vi "Read database.vi"(5 "String":string) -> (0 "error out":errorcluster, 1 "Operator code":string[](array[string]), 2 "DB Data":T1)   [LabVIEW 2015]
uses:
  <vilib>/addons/database/Connection.llb/DB Tools Open Connec (String).vi
  Galobal variable_TI.vi
  <vilib>/addons/database/_DB Variant To Data/Database Variant To Data.xnode
  <vilib>/addons/database/NI_Database_API.lvlib
panel:
  out "data":string[](array[string])
  out "String 2":string
  out "tables":string[](array[string])
  out "error out 3":errorcluster
  out "appended array 4":string[](array[string])
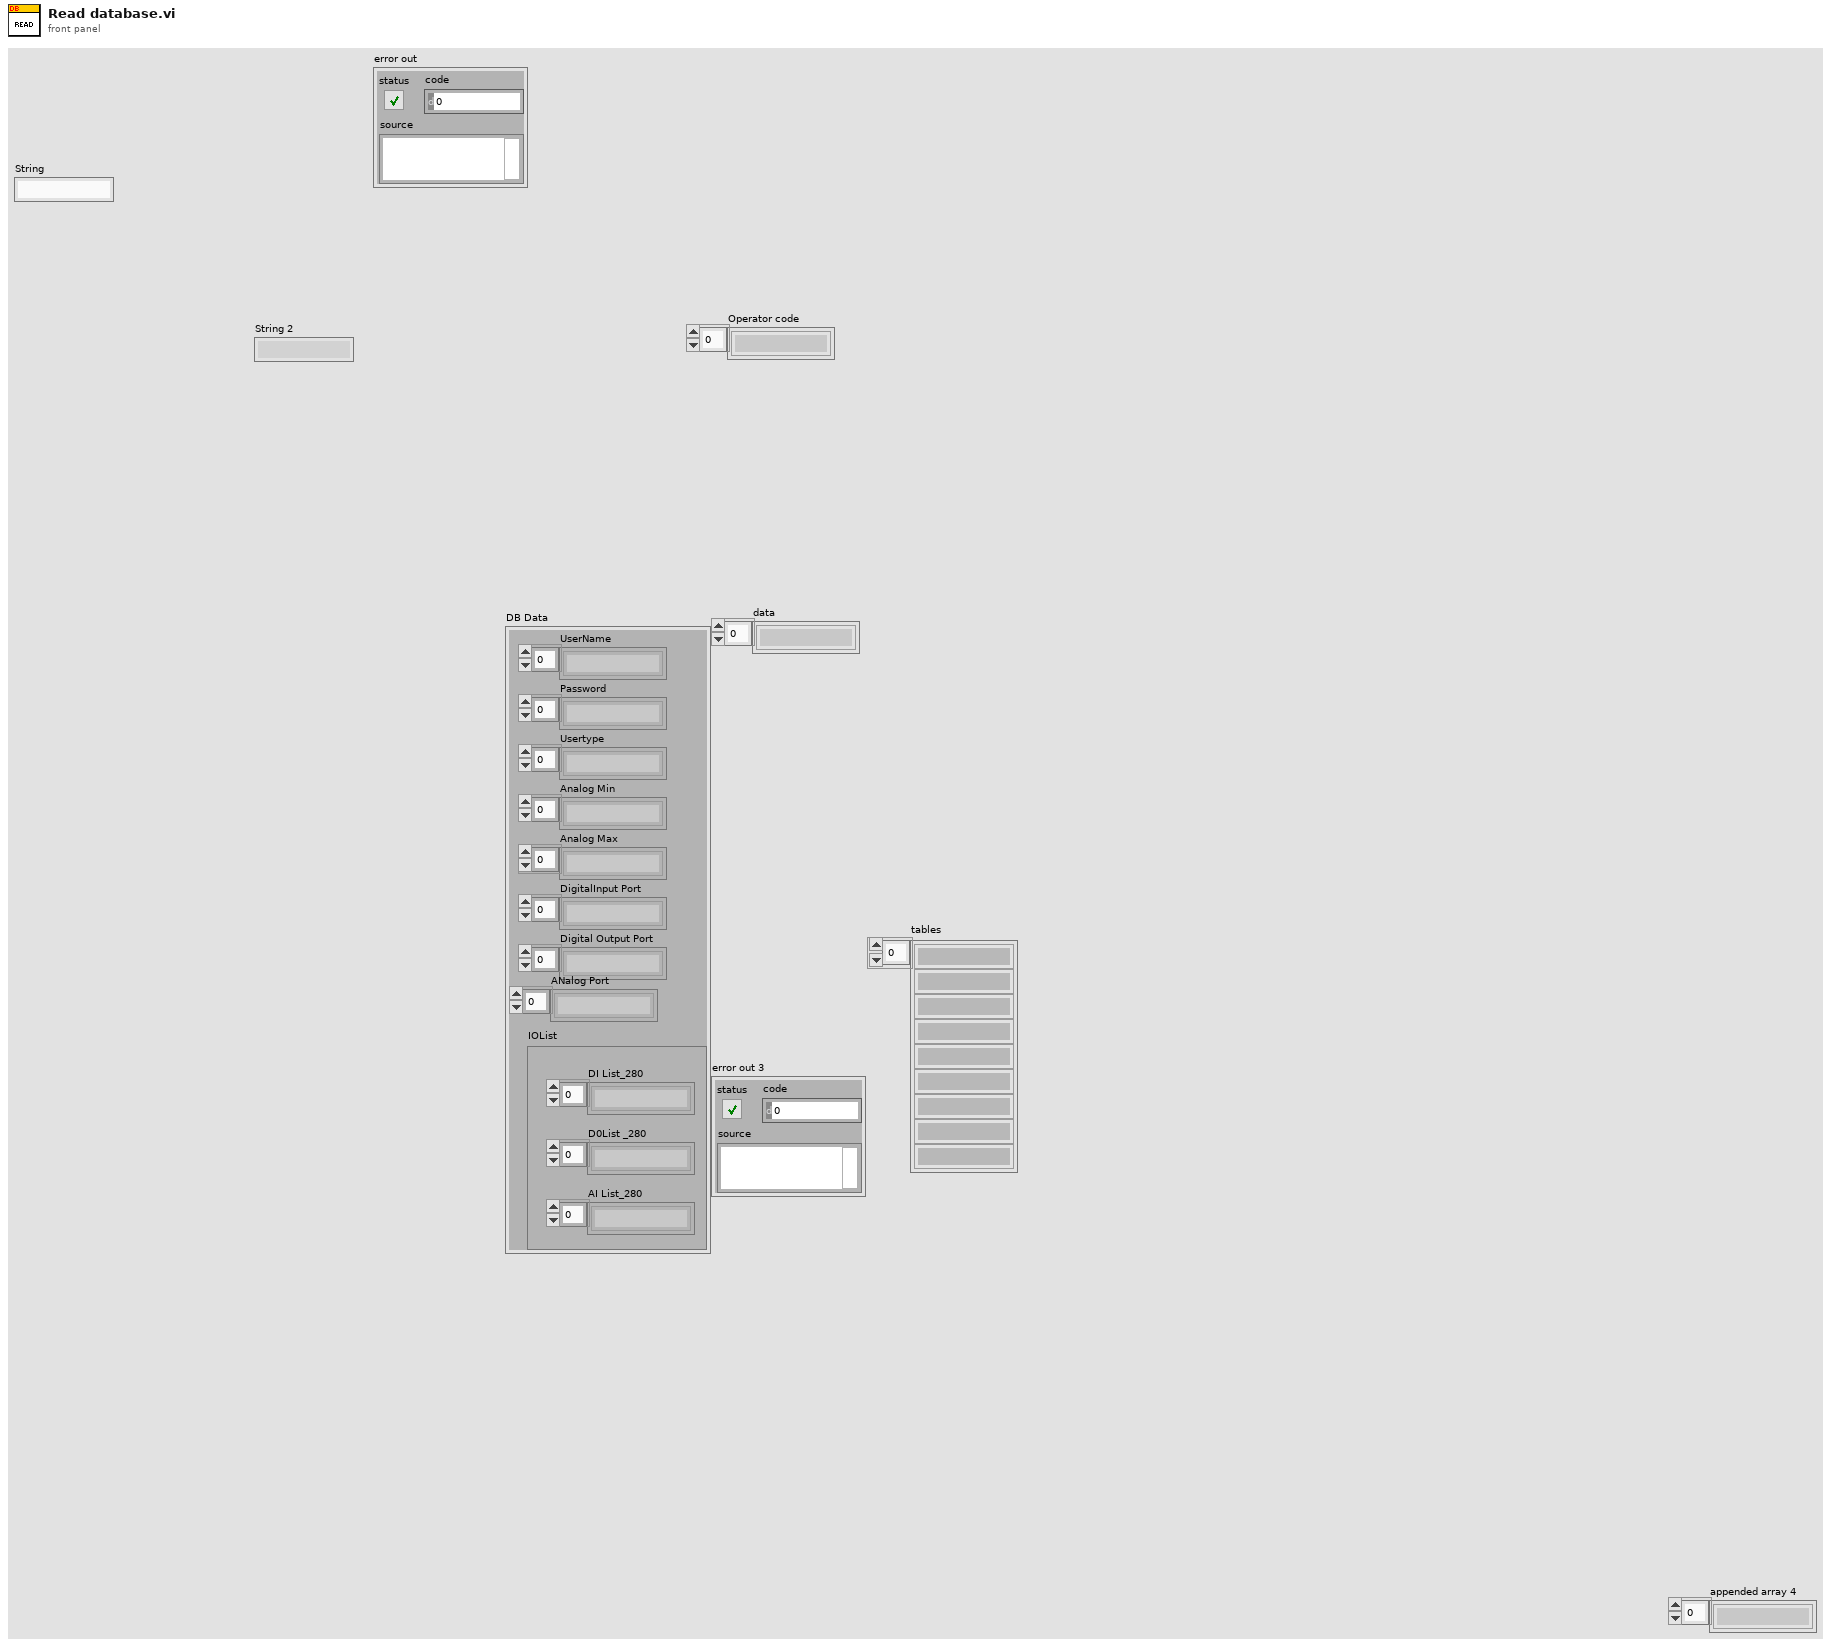
[diagram p1: front panel]
types:
  T1 = cluster{"UserName":string[], "Password":string[], "Usertype":string[], "Analog Min":string[], "Analog Max":string[], "DigitalInput Port":string[], "Digital Output Port":string[], "ANalog Port":string[], "IOList":cluster{"DI List_280":string[], "D0List _280":string[], "AI List_280":string[]}}
  T2 = cluster{"To-A":timestamp, "From-A":timestamp, "From-B":timestamp, "To-B":timestamp, "From-C 1":timestamp, "To-C 1":timestamp, "From-C 2":timestamp, "To-C 2":timestamp, "Shift":string}[]
  T3 = typedef "NI_Database_API.lvlib/Conn ObjectReference.ctl" = refnum<k1>
  T4 = cluster{"DI List_280":string[], "D0List _280":string[], "AI List_280":string[]}
  T5 = cluster{"To-A":timestamp, "From-A":timestamp, "From-B":timestamp, "To-B":timestamp, "From-C 1":timestamp, "To-C 1":timestamp, "From-C 2":timestamp, "To-C 2":timestamp, "Shift":string}
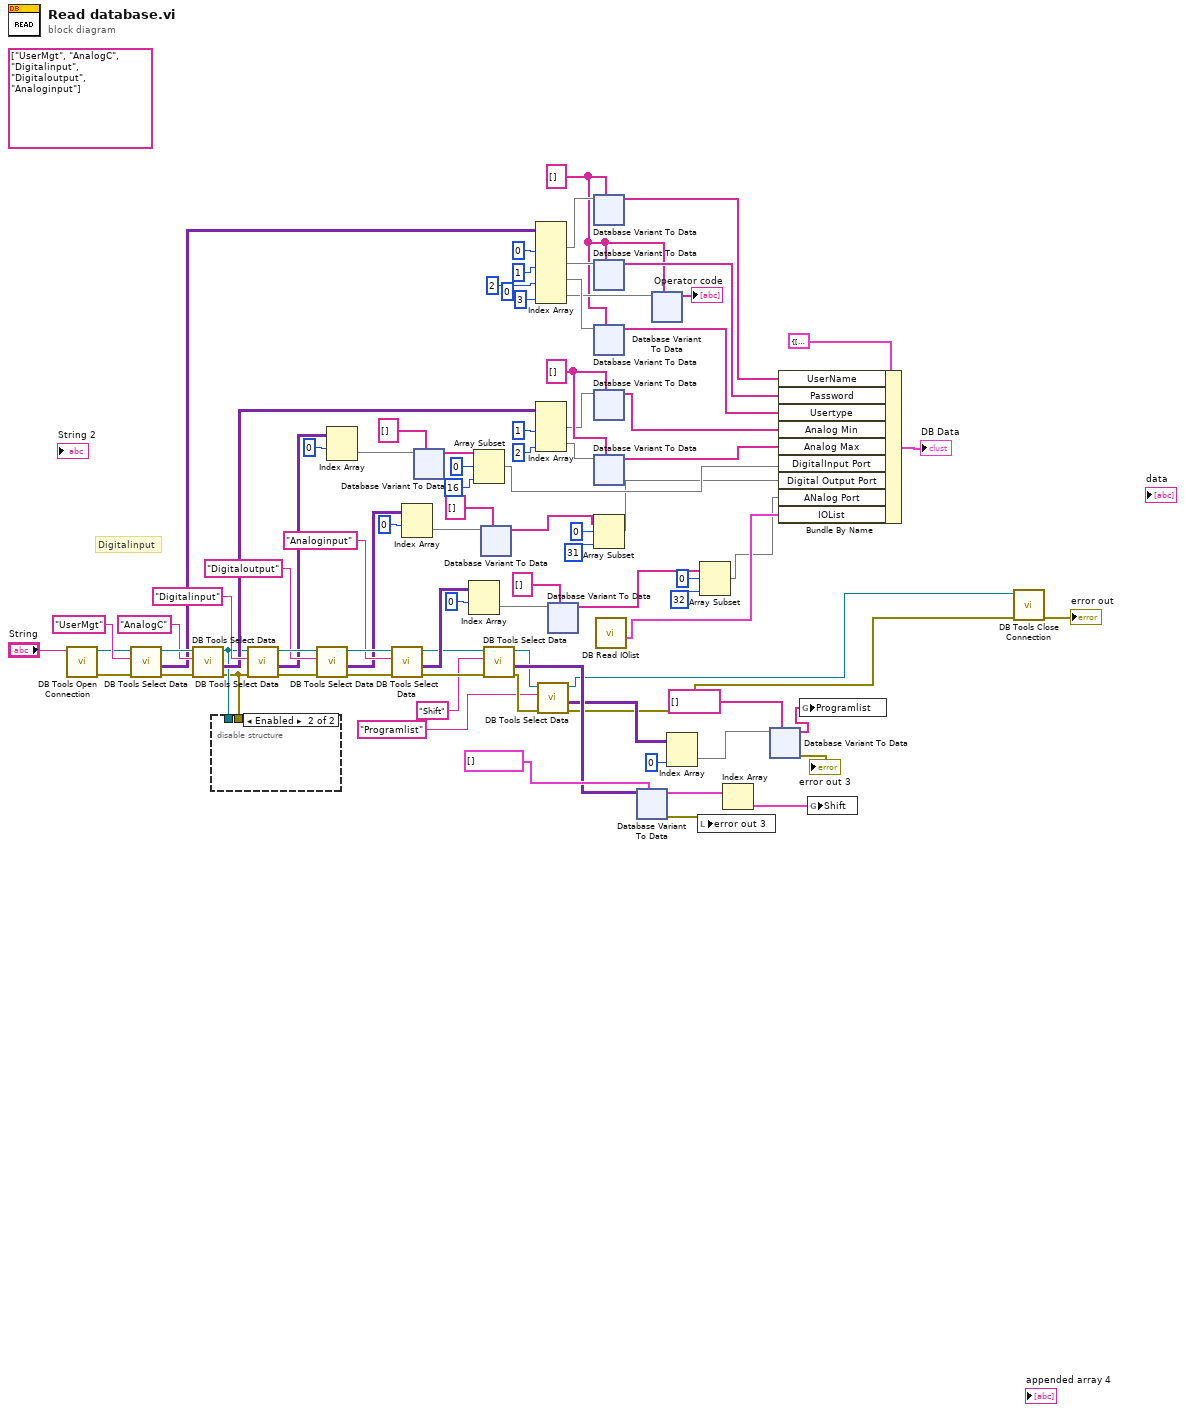
[diagram p0: block diagram]
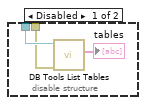
[diagram p2: hidden frame]
diagram:
  (unwired) 0 ("disabled index (row)")
  w76 = string[] []
  (unwired) string[] ["UserMgt", "AnalogC", "Digitalinput", "Digitaloutput", "Analoginput"]
  w2 = string[] []
  # "Digitalinput"
  n1 = call-poly <vilib>:"DB Tools Open Connection.vi"("connection information"="String") -> ("error out"=w46:errorcluster, "connection reference"=w47:T3)  [unwired: 7 in]
  n2 = call <vilib>:"DB Tools Select Data.vi"("error in (no error)"=w46, "table"="UserMgt", "connection reference"=w47) -> ("error out"=w58:errorcluster, "data"=w45:variant[][], "connection reference out"=w57:T3)  [unwired: 3 in]
  n3 = call <vilib>:"DB Tools Select Data.vi"("error in (no error)"=w58, "table"="AnalogC", "connection reference"=w57) -> ("error out"=w8:errorcluster, "data"=w44:variant[][], "connection reference out"=w9:T3)  [unwired: 3 in]
  n4 = disable-structure shown="Enabled" {
    disable-tunnel: w9 -> [w88 _]
    disable-tunnel: w8 -> [w87 _]
    frame Disabled {
      n5 = call <vilib>:"DB Tools List Tables.vi"("error in (no error)"=w87, "connection reference"=w88) -> ("tables"=→"tables":string[])  [unwired: 3 in, 2 out]
    }
    frame Enabled {
    }
  }
  n6 = call <vilib>:"DB Tools Select Data.vi"("error in (no error)"=w8, "table"="Digitalinput", "connection reference"=w9) -> ("error out"=w53:errorcluster, "data"=w43:variant[][], "connection reference out"=w52:T3)  [unwired: 3 in]
  n7 = call <vilib>:"DB Tools Select Data.vi"("error in (no error)"=w53, "table"="Digitaloutput", "connection reference"=w52) -> ("error out"=w49:errorcluster, "data"=w42:variant[][], "connection reference out"=w50:T3)  [unwired: 3 in]
  n8 = Index Array(array=w43, index (row)=0 ("disabled index (col)")) -> (element=w78:variant[])  [unwired: 1 in]
  n9 = call <vilib>:"DB Tools Select Data.vi"("error in (no error)"=w49, "table"="Analoginput", "connection reference"=w50) -> ("error out"=w36:errorcluster, "data"=w41:variant[][], "connection reference out"=w35:T3)  [unwired: 3 in]
  n10 = Index Array(array=w42, index (row)=0 ("disabled index (col)")) -> (element=w79:variant[])  [unwired: 1 in]
  n11 = xnode "Database Variant To Data"("database variant"=w78, "type"=string[] []) -> ("data"=w32:string[])  [unwired: 1 in, 1 out]
  n12 = Index Array(array=w41, index (row)=0 ("disabled index (col)")) -> (element=w82:variant[])  [unwired: 1 in]
  n13 = Array Subset(array=w32, index=0, length=16) -> (w29:string[])
  n14 = xnode "Database Variant To Data"("database variant"=w79, "type"=string[] []) -> ("data"=w27:string[])  [unwired: 1 in, 1 out]
  n15 = call <vilib>:"DB Tools Select Data.vi"("error in (no error)"=w36, "table"="Shift", "connection reference"=w35) -> ("error out"=w19:errorcluster, "data"=w33:variant[][], "connection reference out"=w20:T3)  [unwired: 3 in]
  n16 = Index Array(array=w45, index (col) #1=0 ("disabled index (col)"), index (col) #2=1 ("index (col)"), index (col) #3=2 ("index (col)"), index (col) #4=3 ("index (col)")) -> (element #1=w69:variant[], element #2=w66:variant[], element #3=w65:variant[], element #4=w3:variant[])  [unwired: 4 in]
  n17 = Index Array(array=w44, index (col) #1=1 ("disabled index (col)"), index (col) #2=2 ("index (col)")) -> (element #1=w74:variant[], element #2=w75:variant[])  [unwired: 2 in]
  n18 = call <vilib>:"DB Tools Select Data.vi"("error in (no error)"=w19, "table"="Programlist", "connection reference"=w20) -> ("error out"=w6:errorcluster, "data"=w17:variant[][], "connection reference out"=w7:T3)  [unwired: 3 in]
  n19 = xnode "Database Variant To Data"("database variant"=w82, "type"=string[] []) -> ("data"=w22:string[])  [unwired: 1 in, 1 out]
  n20 = xnode "Database Variant To Data"("database variant"=w69, "type"=w2) -> ("data"=w64:string[])  [unwired: 1 in, 1 out]
  n21 = xnode "Database Variant To Data"("database variant"=w66, "type"=w2) -> ("data"=w63:string[])  [unwired: 1 in, 1 out]
  n22 = xnode "Database Variant To Data"("database variant"=w65, "type"=w2) -> ("data"=w62:string[])  [unwired: 1 in, 1 out]
  n23 = xnode "Database Variant To Data"("database variant"=w74, "type"=w76) -> ("data"=w61:string[])  [unwired: 1 in, 1 out]
  n24 = xnode "Database Variant To Data"("database variant"=w75, "type"=w76) -> ("data"=w60:string[])  [unwired: 1 in, 1 out]
  n25 = Array Subset(array=w27, index=0, length=31) -> (w25:string[])
  n26 = call "DB Read IOlist.vi"() -> ("output cluster"=w21:T4)  [unwired: 11 in]
  n27 = xnode "Database Variant To Data"("database variant"=w33, "type"=T2 []) -> ("data"=w37:T2, "error out"=w10:errorcluster)  [unwired: 1 in]
  n28 = xnode "Database Variant To Data"("database variant"=w3, "type"=w2) -> ("data"=→"Operator code":string[])  [unwired: 1 in, 1 out]
  n29 = Index Array(array=w17, index (col)=0 ("disabled index (col)")) -> (element=w16:variant[])  [unwired: 1 in]
  n30 = local write "error out 3"(w10) -> ()
  n31 = Array Subset(array=w22, index=0, length=32) -> (w12:string[])
  n32 = Index Array(array=w37) -> (element=w5:T5)  [unwired: 1 in]
  n33 = xnode "Database Variant To Data"("database variant"=w16, "type"=string[] []) -> ("data"=w14:string[], "error out"=→"error out 3":errorcluster)  [unwired: 1 in]
  n34 = Bundle By Name(cluster=T1 {"UserName"=[], "Password"=[], "Usertype"=[], "Analog Min"=[], "Analog Max"=[], "DigitalInput Port"=[], "Digital Output Port"=[], "ANalog Port"=[], "IOList"={"DI List_280"=[" Start PB (P0.0) ", "Emergency Stop (P0.1)", "Reset PB (P0.2)", "Home PB (P0.3)", "Main Pressure Signal (P0.4)", "Safety Signal-1 (P0.5)", "Safety Signal-2 (P0.6)", "Fixture Sliding Servo Home RS (P0.7)", "Fixture Sliding Servo Fault Signal (P0.8)", "LCD pressing Servo Home RS (P0.9)", "LCD pressing Servo fault Signal (P0.10)", "Spare", "Spare", "Spare", "Spare", "Model conformation PX-1 (AI2)", "Model conformation PX-2 (AI3)", "Diffuser height checking Sensor-1 (AI4)", "Diffuser height checking Sensor-2 (AI5)", "Panel Door Open Signal (AI6)", "Component CNF Sensor on Ionizer (AI7)", "Bi-adhesive tube Waste Collection bin CNF Sensor (AI8)", "Photo Prism presence Sensor (AI9)", "Lightbox presence CNF Sensor (AI10)", "Diffuser presence CNF Sensor (AI11)", "Photo prism height checking UP CYL Rs (AI12)", "Photo prism height checking DWN CYL  Rs (AI13)", "Camera slide Cyl Fwd Rs (AI14)", "Camera slide Cyl Rev Rs (AI15)", "LCD Display Rotating Unit Actuator Cyl CW PX (AI16)", "LCD Display Rotating Unit Actuator Cyl CCW PX (AI17)", "Fixture clamping Cyl Fwd Rs (AI18)", "Fixture clamping Cyl Rev Rs (AI19)", "Clip pulling unit Cyl Fwd Rs (AI20)", "Clip pulling unit Cyl Rev Rs (AI21)", "Clip clamp unit Cyl Fwd Rs (A22)", "Clip clamp unit Cyl Rev Rs (AI23)", "Barcode Scanner Ready Signal (AI24)", "Spare", "Spare", "Spare", "Spare", "Spare", "Spare", "Spare"], "D0List _280"=["Ionizer ON Sol (P0.16)", "Fixture Slide Servo Fault Reset (P0.17)", "LCD pressing servo Fault Reset (P0.18)", "Fixture Slide servo Brake ON Cmd (P0.19)", "Fixture Slide Servo Direction Command (P0.20)", "LCD pressing Servo Direction Command (P0.21)", "LCD pressing Servo Brake ON Cmd (P0.22)", "Photo prism height checking UP CYL Sol (P0.23)", "Photo prism height checking DWN CYL  Sol (P0.24)", "Camera slide Cyl Fwd Sol (P0.25)", "Camera slide Cyl Rev Sol (P0.26)", "LCD Display Rotating Unit Actuator Cyl CW Sol (P0.27)", "LCD Display Rotating Unit Actuator Cyl CCW Sol (P0.28)", "Fixture clamping Cyl Fwd Sol (P0.29)", "Fixture clamping Cyl Rev Sol (P0.30)", "Clip pulling unit Cyl Fwd Sol (P0.31)", "Clip pulling unit Cyl Rev Sol (P1.0)", "Clip clamp unit Cyl Up Sol (P1.1)", "Clip clamp unit Cyl Dwn Sol (P1.2)", "Optional required based Barcode Trigger Cmd (P1.3)", "TWL Red /Fault with Buzzer (P1.4)", "TWL Green/OK (P1.5)", "TWL Yellow/ Running (P1.6)", "Spare", "Spare", "Spare", "Spare", "Spare", "Fixture Slide Servo Pulse Command (P2.4)", "LCD pressing Servo Pulse Command (P2.5)", "Spare", "Spare"], "AI List_280"=["Loadcell Signal For LCD PRESSING (AI0)", "LVDT SIGNAL FOR PHOTO PRISM HEIGHT CHECK (AI1)"]}} ("DB Data 2"), "UserName"=w64, "Password"=w63, "Usertype"=w62, "Analog Min"=w61, "Analog Max"=w60, "DigitalInput Port"=w29, "Digital Output Port"=w25, "ANalog Port"=w12, "IOList"=w21) -> (→"DB Data":T1)
  n35 = global write "Galobal variable_TI.vi" "Programlist"(w14) -> ()
  n36 = global write "Galobal variable_TI.vi" "Shift"(w5) -> ()
  n37 = call <vilib>:"DB Tools Close Connection.vi"("error in (no error)"=w6, "connection reference"=w7) -> ("error out"=→"error out":errorcluster)  [unwired: 5 in]
